vi "Set_Ramp_rate.vi"(8 "error in (no error)":errorcluster, 10 "New ramp rate":dbl, 11 "Ramper.in":refnum<class "Ramper.lvclass">) -> (0 "error out":errorcluster, 3 "Ramper.out":refnum<class "Ramper.lvclass">)   [LabVIEW 2014, in "Ramper.lvclass"]
uses:
  Ramper.lvclass
  Ramper.lvclass/Ramper.ctl
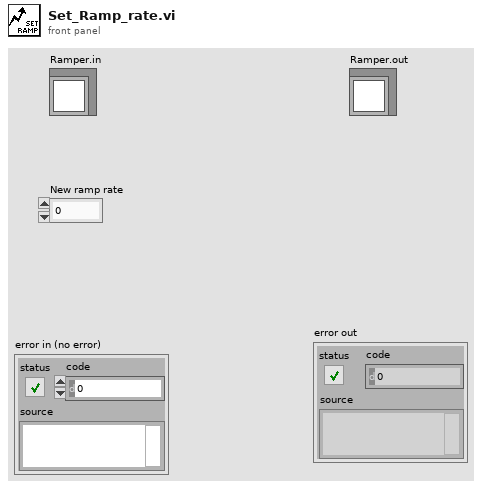
[diagram p1: front panel]
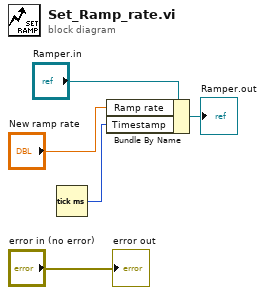
[diagram p0: block diagram]
diagram:
  n1 = Tick Count (ms)() -> (millisecond timer value=w1:u32)
  n2 = Bundle By Name(cluster="Ramper.in", "Ramp rate"="New ramp rate", "Timestamp"=w1) -> (→"Ramper.out":refnum<class "Ramper.lvclass">)
  "error out" <- "error in (no error)"
